vi "ReadServo_R3.vi"(9 "DIO Ref In":T1, 10 "VISA resource name out":refnum<visa-resource-name>, 11 "Servo ID":string="þ") -> (1 "Error":u8, 2 "Valid Checksum":bool=TRUE, 3 "Current Position":u64)   [LabVIEW 2015]
uses:
  <vilib>/myRIO/Instrument Drivers/Onboard IO/DIO/typedefs/DIO Reference.ctl
  <vilib>/myRIO/Common/Instrument Driver Framework/Utilities/typedefs/myRIO Generic Hardware Reference.ctl
  <vilib>/myRIO/Common/Instrument Driver Framework/Utilities/typedefs/Hardware Version Enum.ctl
  <vilib>/myRIO/Common/Instrument Driver Framework/Utilities/typedefs/myRIO v1.0 Reference.ctl
  <vilib>/myRIO/Common/Instrument Driver Framework/Utilities/typedefs/Generic FPGA Reference.ctl
  <vilib>/myRIO/Common/Instrument Driver Framework/myRIO v1.0/DIO/typedefs/DIO Channels List.ctl
  <vilib>/myRIO/Common/Instrument Driver Framework/myRIO v1.0/DIO/typedefs/DIO Channels Enum.ctl
  <vilib>/Utility/error.llb/Error Cluster From Error Code.vi
  <vilib>/myRIO/Common/Instrument Driver Framework/myRIO v1.0/DIO/vis/myRIO v1.0 Write DIO.vi
  <vilib>/myRIO/Instrument Drivers/Onboard IO/DIO/DIO.lvlib
panel:
  out "Calc Cksm":u8
  out "Pre Tx Packet 2":string
  in  "stop":bool
  out "Received\nCksm":u8
  out "Received\nArray":u8[](array[numeric])
  in  "Transmit \nDelay (us)":i32=850
  in  "Return\nDelay (us)":i32=1000
  in  "RECEIVE (F)":bool[](array[boolean])=[FALSE]
  in  "TRANSMIT (T)":bool[](array[boolean])=[TRUE]
  out "Checksum":string="Ó"
  out "Tx Packet":string
  out "Received String Array":string[](array[string])
  out "Received String":string
  # "SEND VALUES"
  # "RECEIVED VALUES"
  # "OUTPUT VALUES"
  # "INPUT"
  # "Config Parameters"
  # "Tx/Rx Delays"
  # "UART HW needs\n1.5-2.5ms to process signal\nkeeping at 2.5ms to be safe"
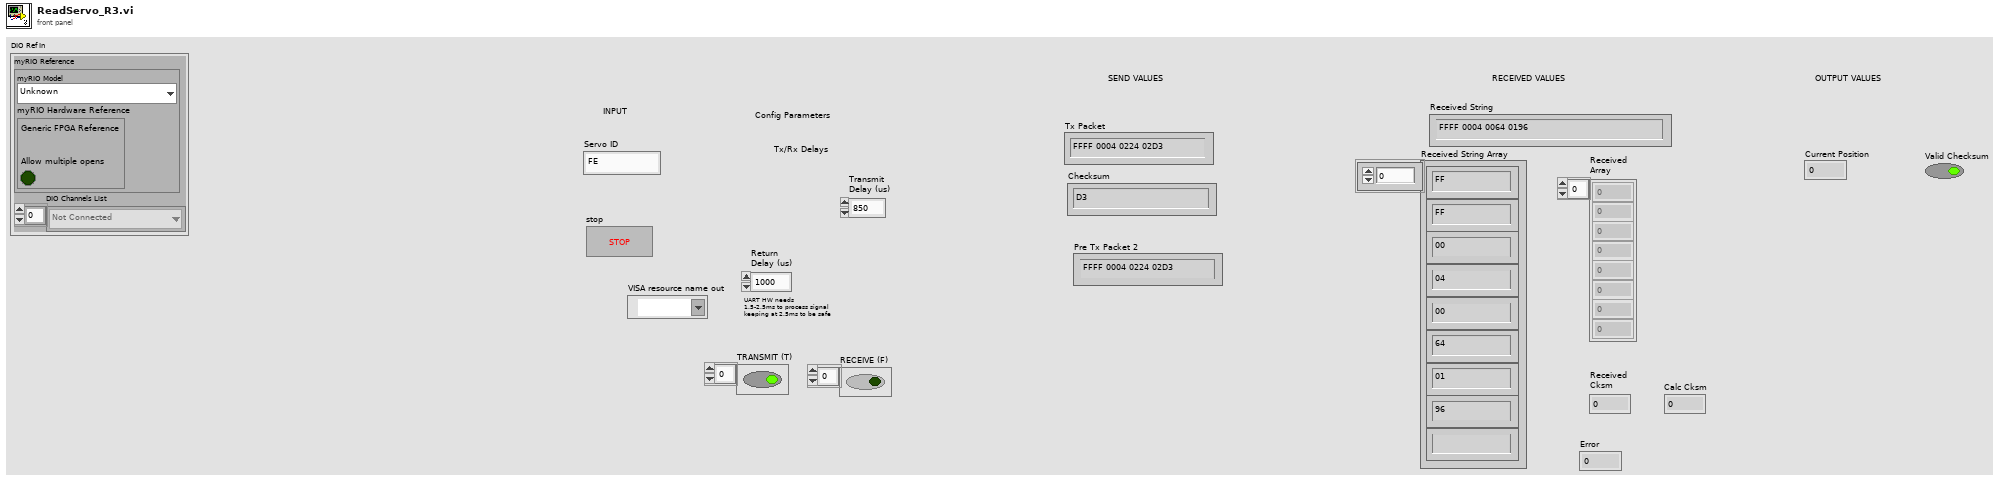
[diagram p1: front panel]
types:
  T1 = typedef "DIO.lvlib/DIO Reference.ctl" = cluster{"myRIO Reference":T2, "DIO Channels List":T6}
  T2 = typedef "myRIO Generic Hardware Reference.ctl" = cluster{"myRIO Model":T3, "myRIO Hardware Reference":T4}
  T3 = typedef "Hardware Version Enum.ctl" = enum16{"Unknown", "myRIO-1900", "myRIO-1950", "roboRIO"}
  T4 = typedef "myRIO v1.0 Reference.ctl" = cluster{"Generic FPGA Reference":T5, "Allow multiple opens":bool}
  T5 = typedef "Generic FPGA Reference.ctl" = refnum<k20>
  T6 = typedef "DIO Channels List.ctl" = T7[]
  T7 = typedef "DIO Channels Enum.ctl" = enum16{"Not Connected", "C/DIO0", "C/DIO1", "C/DIO2", "C/DIO3", "C/DIO4", "C/DIO5", "C/DIO6", "C/DIO7", "A/DIO0", "A/DIO1", "A/DIO2", "A/DIO3", "A/DIO4", "A/DIO5", "A/DIO6", "A/DIO7", "A/DIO8", "A/DIO9", "A/DIO10", "A/DIO11", "A/DIO12", "A/DIO13", "A/DIO14", "A/DIO15", "B/DIO0", "B/DIO1", "B/DIO2", "B/DIO3", "B/DIO4", "B/DIO5", "B/DIO6", "B/DIO7", "B/DIO8", "B/DIO9", "B/DIO10", "B/DIO11", "B/DIO12", "B/DIO13", "B/DIO14", "B/DIO15", "LED0", "LED1", "LED2", "LED3", "Button0", "DIO/DIO0", "DIO/DIO1", "DIO/DIO2", "DIO/DIO3", "DIO/DIO4", "DIO/DIO5", "DIO/DIO6", "DIO/DIO7", "DIO/DIO8", "DIO/DIO9", "SPI/CS0", "SPI/CS1", "SPI/CS2", "SPI/CS3", "LED RADIO (Green)", "LED RADIO (Red)", "LED COMM (Green)", "LED COMM (Red)", "LED MODE (Green)", "LED MODE (Red)"}
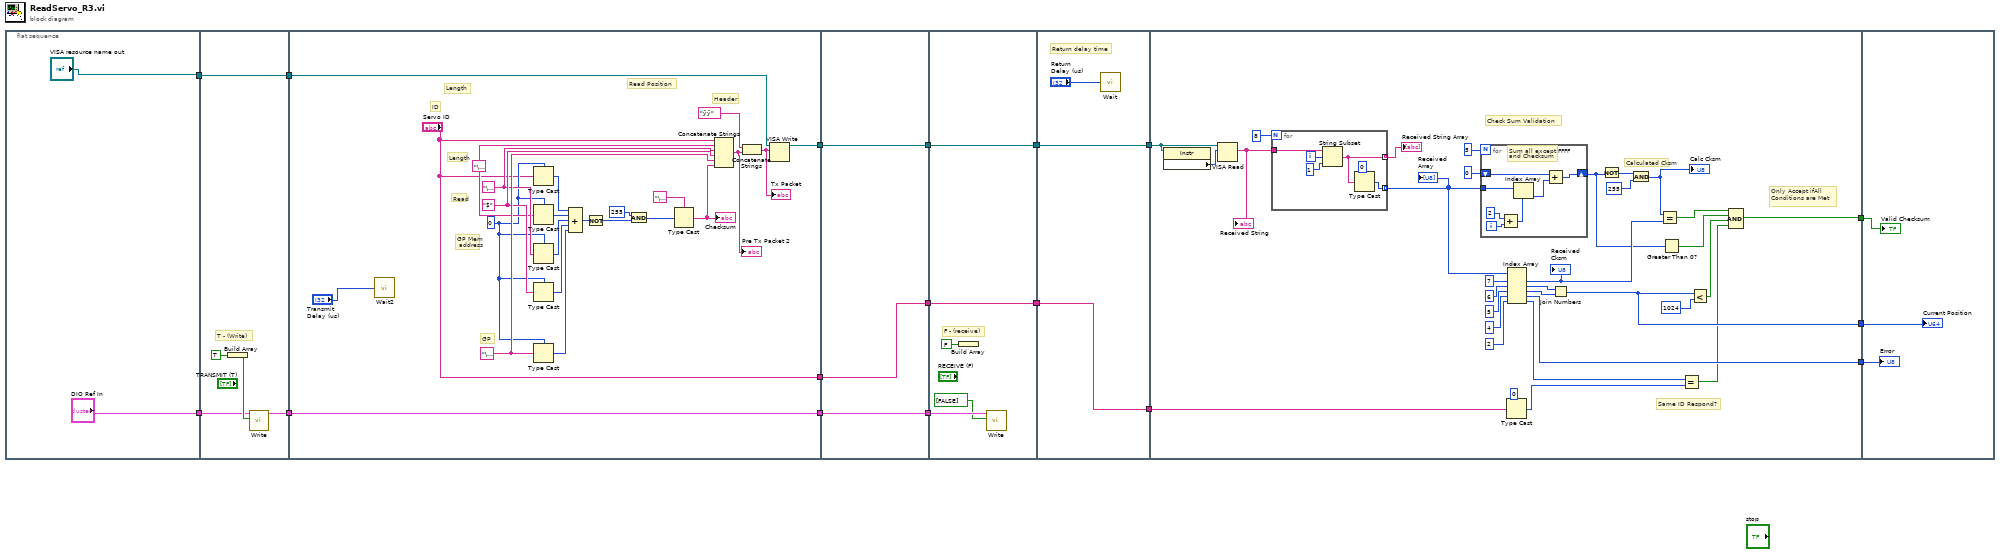
[diagram p0: block diagram]
diagram:
  n1 = flat-sequence {
    tunnel: ["VISA resource name out"] -> w17
    tunnel: ["DIO Ref In"] -> w5
    tunnel: [w24] -> w16
    tunnel: [w22] -> w15
    tunnel: w17 -> [w22]
    tunnel: w5 -> [w20]
    tunnel: [w48] -> w14
    tunnel: [w29] -> w13
    tunnel: ["Servo ID"] -> w2
    tunnel: w15 -> [w31]
    tunnel: w16 -> [w48]
    tunnel: w14 -> [w51]
    tunnel: [w51] -> w12
    tunnel: w13 -> [w50]
    tunnel: [w50] -> w11
    tunnel: [w49] -> w3
    tunnel: w2 -> [w49]
    tunnel: w12 -> [w56]
    tunnel: w11 -> [w54]
    tunnel: [w54] -> w10
    tunnel: [w52] -> w4
    tunnel: w3 -> [w52]
    tunnel: w10 -> [w58]
    tunnel: [w58] -> w9
    tunnel: w4 -> [w57]
    tunnel: [w57] -> w1
    tunnel: w9 -> [w89]
    tunnel: [w60] -> w8
    tunnel: [w70] -> w7
    tunnel: [w72] -> w6
    tunnel: w1 -> [w65]
    tunnel: w8 -> [w107]
    tunnel: w7 -> [w106]
    tunnel: w6 -> [w105]
    frame #0 {
    }
    frame #1 {
      # "T - (Write)"
      n2 = Build Array(TRUE) -> (w21:bool[])
      n3 = call <vilib>:"Write.vi"("Values"=w21, "DIO Ref In"=w20) -> ("DIO Ref Out"=w24:T1)  [unwired: 7 in, 1 out]
    }
    frame #2 {
      w27 = u8 0
      w45 = "$"
      w46 = "\u0002"
      w44 = "\u0002"
      w43 = "\u0004"
      # "Length"
      # "GP Mem\n address"
      # "GP"
      # "Read"
      # "Length"
      # "ID"
      # "Header"
      # "Read Position"
      n4 = call "Wait2"("Count(uSec)"="Transmit \nDelay (us)") -> ()  [unwired: 1 out]
      n5 = Type Cast(type=w27, x="Servo ID") -> (*(type *) &x=w42:u8)
      n6 = Type Cast(type=w27, x=w43) -> (*(type *) &x=w41:u8)
      n7 = Type Cast(type=w27, x=w44) -> (*(type *) &x=w40:u8)
      n8 = Type Cast(type=w27, x=w45) -> (*(type *) &x=w33:u8)
      n9 = Type Cast(type=w27, x=w46) -> (*(type *) &x=w39:u8)
      n10 = Compound Arithmetic op=ADD(w42, w41, w40, w33, w39) -> (w38:u8)
      n11 = Not(x=w38) -> (.not. x?=w36:u8)
      n12 = And(x=u8 255, y=w36) -> (x .and. y?=w34:u8)
      n13 = Type Cast(type="\u0000", x=w34) -> (*(type *) &x=w32:string)
      "Checksum" <- w32
      n14 = Concatenate Strings("Servo ID", w43, w44, w45, w46, w32) -> (w28:string)
      "Pre Tx Packet 2" <- w28
      n15 = Concatenate Strings("ÿÿ", w28) -> (w30:string)
      "Tx Packet" <- w30
      n16 = VISA Write(VISA resource name=w31, write buffer=w30) -> (VISA resource name out=w29:refnum<visa-resource-name>)  [unwired: 1 in, 2 out]
    }
    frame #3 {
    }
    frame #4 {
      # "F - (receive)"
      n17 = Build Array(FALSE) -> ()  [unwired: 1 out]
      n18 = call <vilib>:"Write.vi"("Values"=bool[] [FALSE], "DIO Ref In"=w56) -> ()  [unwired: 7 in, 2 out]
    }
    frame #5 {
      # "Return delay time"
      n19 = call "Wait"("Count(uSec)"="Return\nDelay (us)") -> ()  [unwired: 1 out]
    }
    frame #6 {
      # "Only Accept ifAll\nConditions are Met"
      # "Same ID Respond?"
      # "Calculated Cksm"
      # "Check Sum Validation"
      n20 = property class="Instr"(reference=w89) -> ("Serial Settings:Number of Bytes at Serial Port"=w88:u32)  [unwired: 1 in, 2 out]
      n21 = VISA Read(VISA resource name=w89, byte count=w88) -> (read buffer=w90:string)  [unwired: 1 in, 3 out]
      "Received String" <- w90
      n22 = for {
        N: 8 -> [_]
        tunnel: w90 -> [w104]
        tunnel: [w100] -> w87 mode=indexing
        tunnel: [w99] -> w85 mode=indexing
        i -> [w103]
        n23 = String Subset(string=w104, offset (0)=w103, length (rest)=1) -> (substring=w100:string)
        n24 = Type Cast(type=u8 0, x=w100) -> (*(type *) &x=w99:u8)
      }
      "Received String Array" <- w87
      "Received\nArray" <- w85
      n25 = for {
        N: 5 -> [_]
        tunnel: w85 -> [w95]
        shift-right: [w94] -> w74
        shift-left: u8 0 -> [w93]
        i -> [w98]
        # "Sum all except FFFF\nand Checksum"
        n26 = Add(x=2, y=w98) -> (x+y=w96:i32)
        n27 = Index Array(array=w95, index=w96) -> (element=w92:u8)
        n28 = Add(x=w93, y=w92) -> (x+y=w94:u8)
      }
      n29 = Type Cast(type=u8 0, x=w65) -> (*(type *) &x=w68:u8)
      n30 = Index Array(array=w85, index #1=7 ("x"), index #2=6 ("x"), index #3=5 ("x"), index #4=4 ("x"), index #5=2 ("x")) -> (element #1=w79:u8, element #2=w76:u8, element #3=w75:u8, element #4=w72:u8, element #5=w66:u8)
      "Received\nCksm" <- w79
      n31 = Join Numbers(hi=w76, lo=w75) -> ((hi.lo)=w70:u16)
      n32 = Not(x=w74) -> (.not. x?=w82:u8)
      n33 = And(x=w82, y=u8 255) -> (x .and. y?=w80:u8)
      "Calc Cksm" <- w80
      n34 = Equal?(x=w80, y=w79) -> (x = y?=w64:bool)
      n35 = Greater Than 0?(x=w74) -> (x > 0?=w63:bool)
      n36 = Equal?(x=w66, y=w68) -> (x = y?=w61:bool)
      n37 = Less?(x=w70, y=u16 1024) -> (x < y?=w62:bool)
      n38 = Compound Arithmetic op=AND(w64, w63, w62, w61) -> (w60:bool)
    }
    frame #7 {
      "Valid Checksum" <- w107
      "Current Position" <- w106
      "Error" <- w105
    }
  }
